vi "get data type.vi"(8 "error in (no error)":errorcluster, 11 "data array":string[](array[string])) -> (0 "error out":errorcluster, 3 "data type":string[](array[string]))   [LabVIEW 2019]
uses:
  <vilib>/JDP Science/JSONtext/JSONtext.lvlib
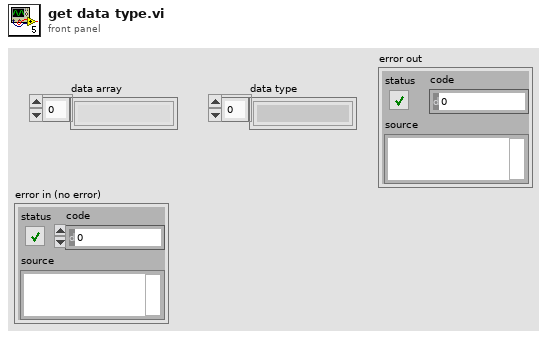
[diagram p1: front panel]
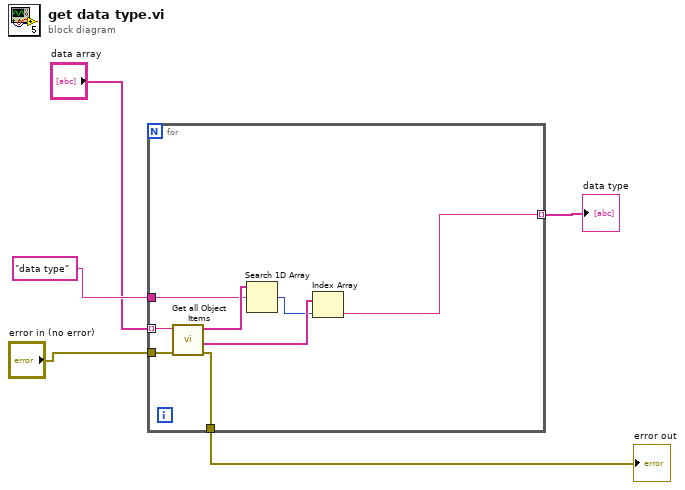
[diagram p0: block diagram]
diagram:
  n1 = for {
    tunnel: "data array" -> [w13] mode=indexing
    tunnel: [w6] -> w3 mode=indexing
    tunnel: "data type" ("Search type") -> [w9]
    tunnel: "error in (no error)" -> [w8]
    tunnel: [w7] -> w4
    n2 = call <vilib>:"Get all Object Items.vi"("error in (no error)"=w8, "JSON"=w13) -> ("error out"=w7:errorcluster, "<JSON>"=w12:string[], "Item Names"=w10:string[])  [unwired: 6 in, 1 out]
    n3 = Search 1D Array(1D array=w10, element=w9) -> (index of element=w11:i32)  [unwired: 1 in]
    n4 = Index Array(array=w12, index=w11) -> (element=w6:string)
  }
  "data type" <- w3
  "error out" <- w4
